vi "AODO-Wait To Write (new).vi"(0 "Tnext in":dbl format="%#_16g", 2 "Headway":dbl, 11 "error in (no error)":errorcluster, 12 "Frame size":i32, 13 "Poll (s)":dbl) -> (4 "Tnext out":dbl format="%#_16g", 15 "error out":errorcluster)   [LabVIEW 2020]
uses:
  Typedefs/AODO-Action.ctl
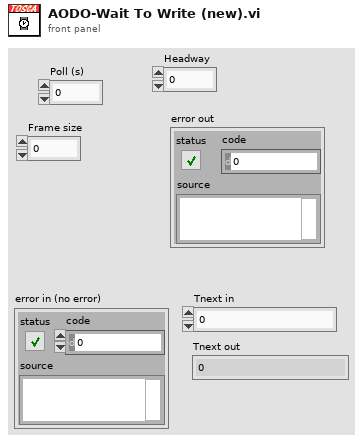
[diagram p1: front panel]
types:
  T1 = typedef "AODO-Action.ctl" = enum16{"Configure", "Initialize", "Start", "Write", "Clean up", "Init & Start", "Config & Test", "Position", "Set AO Gains", "Zero"}
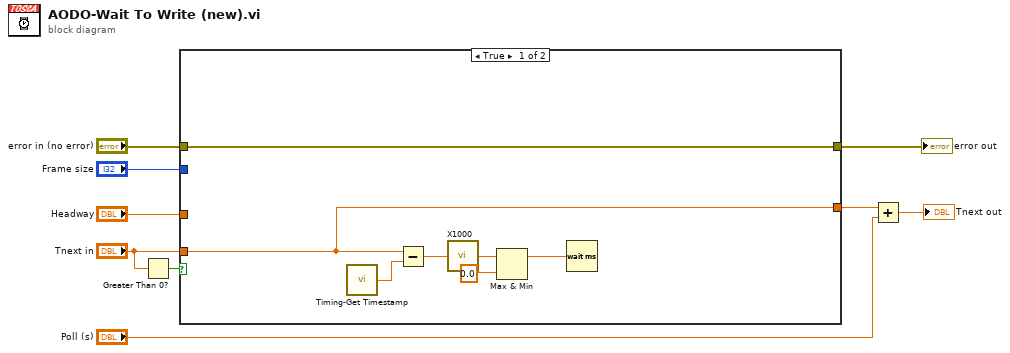
[diagram p0: block diagram]
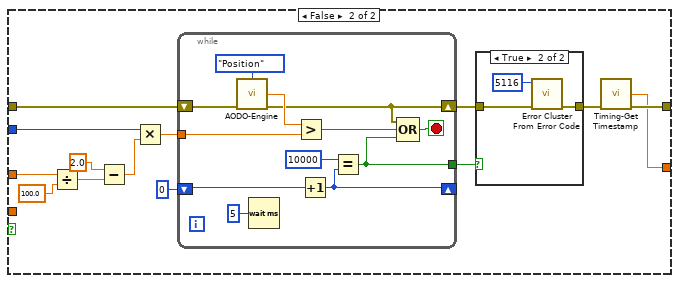
[diagram p2: hidden frame]
diagram:
  n1 = Greater Than 0?(x="Tnext in") -> (x > 0?=w4:bool)
  n2 = case shown="True" w4 {
    tunnel: [w12 w26] -> w8
    tunnel: "error in (no error)" -> [w12 w28]
    tunnel: [w14 w25] -> w5
    tunnel: "Tnext in" -> [w14 _]
    tunnel: "Frame size" -> [_ w20]
    tunnel: "Headway" -> [_ w19]
    frame True {
      n3 = call "Timing-Get Timestamp.vi"() -> ("double precision float"=w10:dbl)  [unwired: 14 in, 1 out]
      n4 = Subtract(x=w14, y=w10) -> (x-y=w16:dbl)
      n5 = call "X1000.vi"("X"=w16) -> ("X/1000"=w15:dbl)
      n6 = Max & Min(x=w15, y=0.0) -> (max(x,y)=w11:dbl)  [unwired: 1 out]
      n7 = Wait (ms)(milliseconds to wait=w11) -> ()  [unwired: 1 out]
    }
    frame False {
      n8 = Divide(x=w19, y=100.0) -> (x/y=w18:dbl)
      n9 = Subtract(x=2.0, y=w18) -> (x-y=w22:dbl)
      n10 = Multiply(x=w20, y=w22) -> (x*y=w21:dbl)
      n11 = while {
        tunnel: w21 -> [w44]
        shift-right: [w39] -> _
        shift-left: 0 -> [w40]
        tunnel: [w37] -> w30
        shift-right: [w43] -> w29
        shift-left: w28 -> [w36]
        stop <- w41 stop-if-true
        n12 = call "AODO-Engine.vi"("Action"=AODO-Action."Position", "error in (no error)"=w36) -> ("Position"=w45:dbl, "error out"=w43:errorcluster)  [unwired: 9 in, 3 out]
        n13 = Wait (ms)(milliseconds to wait=u32 5) -> ()  [unwired: 1 out]
        n14 = Greater?(x=w45, y=w44) -> (0:w42:bool)
        n15 = Increment(x=w40) -> (x+1=w39:i32)
        n16 = Equal?(x=10000, y=w39) -> (x = y?=w37:bool)
        n17 = Compound Arithmetic op=OR(w43, w42, w37) -> (w41:bool)
      }
      n18 = case shown="True" w30 {
        tunnel: w29 -> [w31 w34]
        tunnel: [w31 w33] -> w27
        frame False {
        }
        frame True {
          n19 = call <vilib>:"Error Cluster From Error Code.vi"("error in (no error)"=w34, "error code (0)"=5116) -> ("error out"=w33:errorcluster)  [unwired: 7 in]
        }
      }
      n20 = call "Timing-Get Timestamp.vi"("error in (no error)"=w27) -> ("double precision float"=w25:dbl, "error out"=w26:errorcluster)  [unwired: 13 in]
    }
  }
  "error out" <- w8
  n21 = Add(x=w5, y="Poll (s)") -> (x+y=→"Tnext out":dbl)
